vi "WSVCAP SHL Host LL I2C Build DUT Mask.vi"(0 "DUT":T1) -> (4 "Socket Mask [U64]":u64 format="%016x", 8 "DUT Mask":bool[](array[boolean]))   [LabVIEW 2017]
uses:
  Type Defs/WSVCAP SHL DUT Number Enum.ctl
panel:
  # "DUT 01"
  # "DUT 02"
  # "DUT 03"
  # "DUT 04"
  # "DUT 05"
  # "DUT 06"
  # "DUT 07"
  # "DUT 08"
  # "DUT 09"
  # "DUT 10"
  # "DUT 11"
  # "DUT 12"
  # "DUT 13"
  # "DUT 14"
  # "DUT 15"
  # "DUT 16"
  # "DUT 17"
  # "DUT 18"
  # "DUT 19"
  # "DUT 20"
  # "DUT 21"
  # "DUT 22"
  # "DUT 23"
  # "DUT 24"
  # "DUT 25"
  # "DUT 26"
  # "DUT 27"
  # "DUT 28"
  # "DUT 29"
  # "DUT 30"
  # "DUT 31"
  # "DUT 32"
  # "DUT 33"
  # "DUT 34"
  # "DUT 35"
  # "DUT 36"
  # "DUT 37"
  # "DUT 38"
  # "DUT 39"
  # "DUT 40"
  # "DUT 41"
  # "DUT 42"
  # "DUT 43"
  # "DUT 44"
  # "DUT 45"
  # "DUT 46"
  # "DUT 47"
  # "DUT 48"
  # "DUT 49"
  # "DUT 50"
  # "DUT 51"
  # "DUT 52"
  # "DUT 53"
  # "DUT 54"
  # "DUT 55"
  # "DUT 56"
  # "DUT 57"
  # "DUT 58"
  # "DUT 59"
  # "DUT 60"
  # "DUT 61"
  # "DUT 62"
  # "DUT 63"
  # "DUT 64"
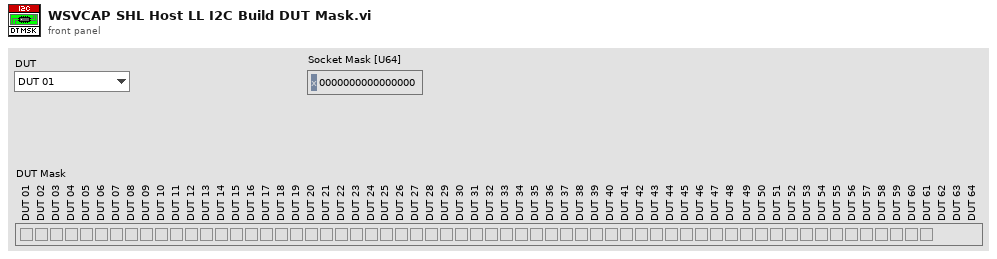
[diagram p1: front panel]
types:
  T1 = typedef "WSVCAP SHL DUT Number Enum.ctl" = enum16{"DUT 01", "DUT 02", "DUT 03", "DUT 04", "DUT 05", "DUT 06", "DUT 07", "DUT 08", "DUT 09", "DUT 10", "DUT 11", "DUT 12", "DUT 13", "DUT 14", "DUT 15", "DUT 16", "DUT 17", "DUT 18", "DUT 19", "DUT 20", "DUT 21", "DUT 22", "DUT 23", "DUT 24", "DUT 25", "DUT 26", "DUT 27", "DUT 28", "DUT 29", "DUT 30", "DUT 31", "DUT 32", "DUT 33", "DUT 34", "DUT 35", "DUT 36", "DUT 37", "DUT 38", "DUT 39", "DUT 40", "DUT 41", "DUT 42", "DUT 43", "DUT 44", "DUT 45", "DUT 46", "DUT 47", "DUT 48", "DUT 49", "DUT 50", "DUT 51", "DUT 52", "DUT 53", "DUT 54", "DUT 55", "DUT 56", "DUT 57", "DUT 58", "DUT 59", "DUT 60", "DUT 61", "DUT 62", "DUT 63", "DUT 64"}
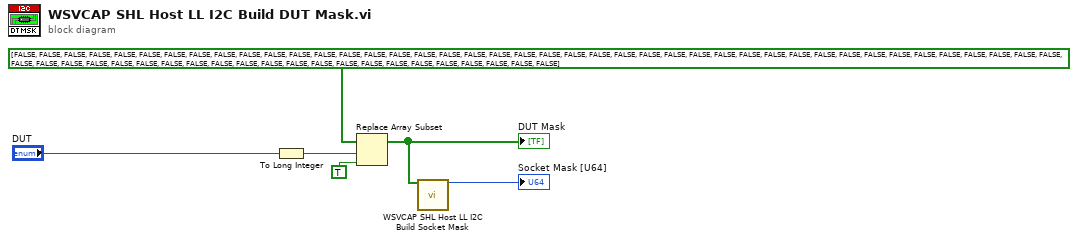
[diagram p0: block diagram]
diagram:
  n1 = To Long Integer(number="DUT") -> (32bit integer=w1:i32)
  n2 = Replace Array Subset(array=bool[] [FALSE, FALSE, FALSE, FALSE, FALSE, FALSE, FALSE, FALSE, FALSE, FALSE, FALSE, FALSE, FALSE, FALSE, FALSE, FALSE, FALSE, FALSE, FALSE, FALSE, FALSE, FALSE, FALSE, FALSE, FALSE, FALSE, FALSE, FALSE, FALSE, FALSE, FALSE, FALSE, FALSE, FALSE, FALSE, FALSE, FALSE, FALSE, FALSE, FALSE, FALSE, FALSE, FALSE, FALSE, FALSE, FALSE, FALSE, FALSE, FALSE, FALSE, FALSE, FALSE, FALSE, FALSE, FALSE, FALSE, FALSE, FALSE, FALSE, FALSE, FALSE, FALSE, FALSE, FALSE], new element=TRUE, index=w1) -> (w5:bool[])
  "DUT Mask" <- w5
  n3 = call "WSVCAP SHL Host LL I2C Build Socket Mask.vi"("DUT Mask Array"=w5) -> ("Socket Mask Set [U64]"=→"Socket Mask [U64]":u64)  [unwired: 14 in]
